vi "Factor multiply.vi"(4 "factor":sgl, 6 "Numeric IN":sgl) -> (1 "Numeric OUT":sgl)   [LabVIEW 2012]
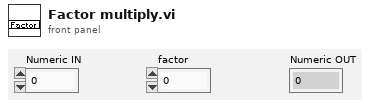
[diagram p1: front panel]
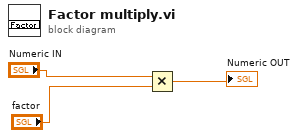
[diagram p0: block diagram]
diagram:
  n1 = Multiply(x="Numeric IN", y="factor") -> (x*y=→"Numeric OUT":sgl)
